vi "FGV.vi"(8 "error in (no error)":errorcluster, 10 "FGV_State":T1) -> (0 "error out":errorcluster, 3 "FGV":T2 {"Database"."Balance" format="%#.2f"; "Database"."Account Number" format="%_1f"})   [LabVIEW 2020]
doc: "FGV is used to manage all data configuration as Events ref , Queue message handling ref and DB (Read / update)"
uses:
  Controls/FGV_Data.ctl
  SubVIs/Message Queue/All Message Queues.ctl
  SubVIs/Message Queue/Message Cluster.ctl
  Controls/Events_User.ctl
  Database/Controls/Account Database.ctl
  Controls/FGV_State.ctl
  Database/Controls/Todo.ctl
  Controls/Data_Initialize.ctl
  SubVIs/User Event - Stop/User Event - Stop.lvlib
  SubVIs/Message Queue/Message Queue.lvlib
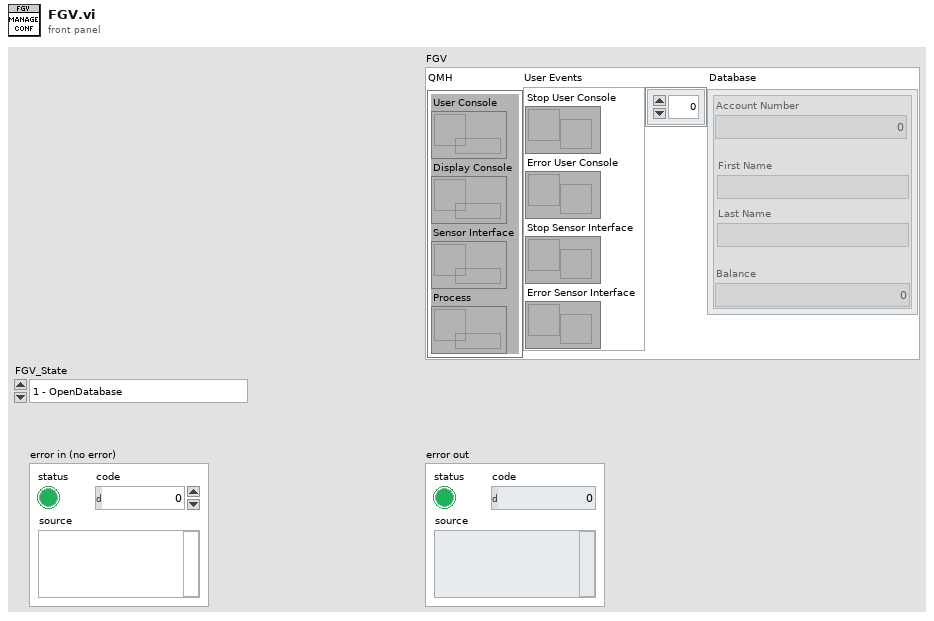
[diagram p1: front panel]
types:
  T1 = typedef "FGV_State.ctl" = enum16{"1 - OpenDatabase", "2 - Initialize Events", "3 - Initialize QMH", "4 - Close QMH", "5 - Close Events", "Read FGV", "Save Database", "Def"}
  T2 = typedef "FGV_Data.ctl" = cluster{"QMH":T3, "User Events":T4, "Database":T5[]}
  T3 = typedef "Message Queue.lvlib/All Message Queues.ctl" = cluster{"User Console":refnum<queue>, "Display Console":refnum<queue>, "Sensor Interface":refnum<queue>, "Process":refnum<queue>}
  T4 = typedef "Events_User.ctl" = cluster{"Stop User Console":refnum<user-event>, "Error User Console":refnum<user-event>, "Stop Sensor Interface ":refnum<user-event>, "Error Sensor Interface":refnum<user-event>}
  T5 = typedef "Account Database.ctl" = cluster{"Account Number":i32, "First Name":string, "Last Name":string, "Balance":dbl}
  T6 = typedef "Todo.ctl" = enum16{"Read", "Update"}
  T7 = typedef "Data_Initialize.ctl" = cluster{"Database":T5[], "User Events":T4}
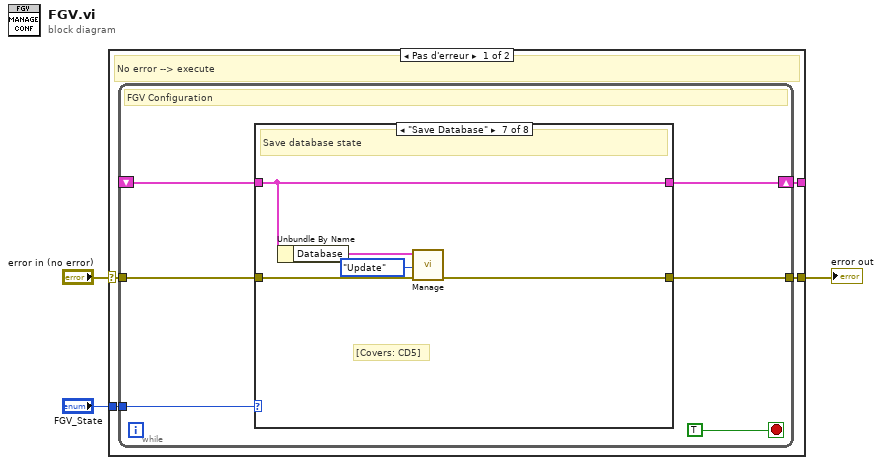
[diagram p0: block diagram]
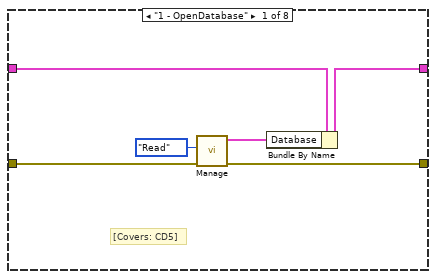
[diagram p2: hidden frame]
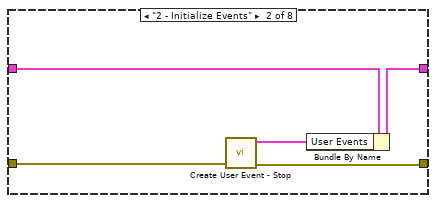
[diagram p3: hidden frame]
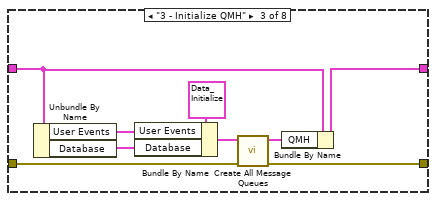
[diagram p4: hidden frame]
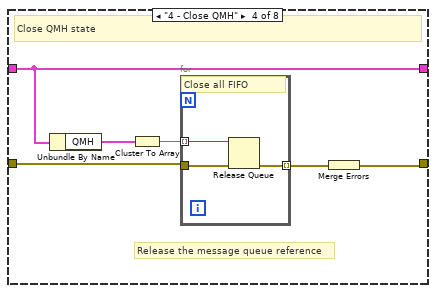
[diagram p5: hidden frame]
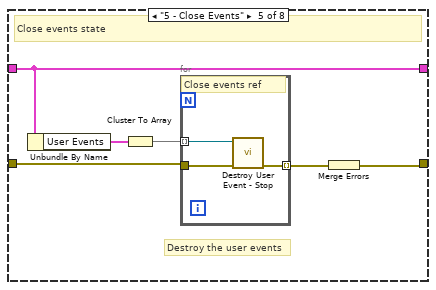
[diagram p6: hidden frame]
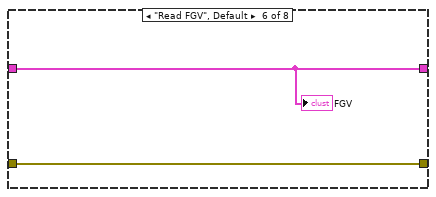
[diagram p7: hidden frame]
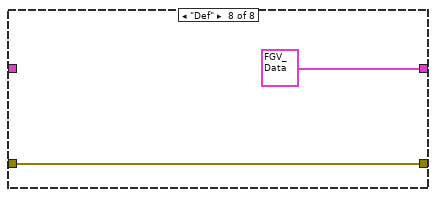
[diagram p8: hidden frame]
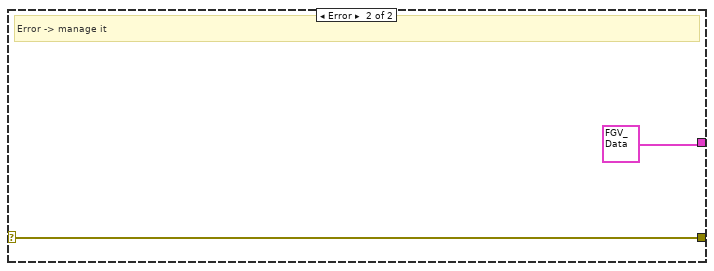
[diagram p9: hidden frame]
diagram:
  n1 = case shown="Pas d'erreur" "error in (no error)" {
    selector: "error in (no error)" -> [w5 w62]
    tunnel: [w7 T2 {"QMH"={"User Console"=refnum, "Display Console"=refnum, "Sensor Interface"=refnum, "Process"=refnum}, "User Events"={"Stop User Console"=refnum, "Error User Console"=refnum, "Stop Sensor Interface "=refnum, "Error Sensor Interface"=refnum}, "Database"=[]} ("FGV 2")] -> _
    tunnel: [w6 w62] -> w3
    tunnel: "FGV_State" -> [w4 _]
    frame No Error {
      # "No error --> execute"
      n2 = while {
        tunnel: w4 -> [w12]
        shift-right: [w10] -> w7
        shift-left: _ -> [w11]
        tunnel: w5 -> [w9]
        tunnel: [w8] -> w6
        stop <- TRUE stop-if-true
        # "FGV Configuration"
        n3 = case shown="\"Save Database\"" w12 {
          tunnel: w11 -> [w19 w22 w27 w38 w47 w52 w58 _]
          tunnel: [w16 w21 w31 w38 w47 w52 w58 T2 {"QMH"={"User Console"=refnum, "Display Console"=refnum, "Sensor Interface"=refnum, "Process"=refnum}, "User Events"={"Stop User Console"=refnum, "Error User Console"=refnum, "Stop Sensor Interface "=refnum, "Error Sensor Interface"=refnum}, "Database"=[]} ("FGV 2")] -> w10
          tunnel: w9 -> [w18 w24 w33 w39 w48 w53 w55 w60]
          tunnel: [w17 w23 w32 w34 w43 w53 w54 w60] -> w8
          frame "1 - OpenDatabase" {
            # "[Covers: CD5]"
            n4 = call "Manage.vi"("error in"=w18, "ToDo"=Todo."Read") -> ("error out"=w17:errorcluster, "Database OUT"=w15:T5[])  [unwired: 8 in]
            n5 = Bundle By Name(cluster=w19, "Database"=w15) -> (w16:T2)
          }
          frame "2 - Initialize Events" {
            n6 = call "Create User Event - Stop.vi"("error in (no error)"=w24) -> ("error out"=w23:errorcluster, "User Events"=w20:T4)  [unwired: 9 in]
            n7 = Bundle By Name(cluster=w22, "User Events"=w20) -> (w21:T2)
          }
          frame "3 - Initialize QMH" {
            n8 = Unbundle By Name(w27) -> ("User Events"=w25:T4, "Database"=w26:T5[])
            n9 = Bundle By Name(cluster=T7 {"Database"=[], "User Events"={"Stop User Console"=refnum, "Error User Console"=refnum, "Stop Sensor Interface "=refnum, "Error Sensor Interface"=refnum}} ("Initiliaze"), "User Events"=w25, "Database"=w26) -> (w28:T7)
            n10 = call "Create All Message Queues.vi"("error in (no error)"=w33, "Initiliaze"=w28) -> ("error out"=w32:errorcluster, "QMH"=w30:T3)  [unwired: 8 in]
            n11 = Bundle By Name(cluster=w27, "QMH"=w30) -> (w31:T2)
          }
          frame "4 - Close QMH" {
            # "Release the message queue reference"
            # "Close QMH state"
            n12 = Unbundle By Name(w38) -> ("QMH"=w37:T3)
            n13 = Cluster To Array(cluster=w37) -> (array=w36:refnum<queue>[])
            n14 = for {
              tunnel: w36 -> [w40] mode=indexing
              tunnel: w39 -> [w42]
              tunnel: [w41] -> w35 mode=indexing
              # "Close all FIFO"
              n15 = Release Queue(queue=w40, error in (no error)=w42) -> (error out=w41:errorcluster)  [unwired: 1 in, 2 out]
            }
            n16 = Merge Errors(w35) -> (w34:errorcluster)
          }
          frame "5 - Close Events" {
            # "Destroy the user events"
            # "Close events state"
            n17 = Unbundle By Name(w47) -> ("User Events"=w46:T4)
            n18 = Cluster To Array(cluster=w46) -> (array=w45:refnum<user-event>[])
            n19 = for {
              tunnel: w45 -> [w51] mode=indexing
              tunnel: w48 -> [w50]
              tunnel: [w49] -> w44 mode=indexing
              # "Close events ref"
              n20 = call "Destroy User Event - Stop.vi"("error in (no error)"=w50, "User Event - Stop"=w51) -> ("error out"=w49:errorcluster)  [unwired: 9 in]
            }
            n21 = Merge Errors(w44) -> (w43:errorcluster)
          }
          frame "Read FGV", Default {
            "FGV" <- w52
          }
          frame "Save Database" {
            # "[Covers: CD5]"
            # "Save database state"
            n22 = Unbundle By Name(w58) -> ("Database"=w57:T5[])
            n23 = call "Manage.vi"("error in"=w55, "ToDo"=Todo."Update", "Database IN"=w57) -> ("error out"=w54:errorcluster)  [unwired: 7 in, 1 out]
          }
          frame "Def" {
          }
        }
      }
    }
    frame Error {
      # "Error -> manage it"
    }
  }
  "error out" <- w3
